vi "Configure Device.vi"(8 "error in (no error)":errorcluster, 11 "Signal Generator in":refnum<class "Signal Generator.lvclass">) -> (0 "error out":errorcluster, 3 "Signal Generator out":refnum<class "Signal Generator.lvclass">)   [LabVIEW 2020, in "Signal Generator.lvlib" / "Signal Generator.lvclass"]
uses:
  Signal Generator.lvclass
  Waveform Type.ctl
  Waveform Definition.ctl
  build/ppl/lv-hal.lvlibp/Device/Device.lvclass
  C:/dev/HAL Demo/build/ppl/lv-hal.lvlibp/Device/Device.lvclass
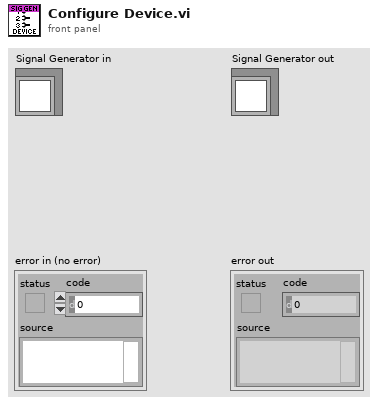
[diagram p1: front panel]
types:
  T1 = typedef "Signal Generator.lvlib/Signal Generator.lvclass/Waveform Definition.ctl" = cluster{"Waveform Type":T2, "Frequency":dbl, "Amplitude":dbl}
  T2 = typedef "Signal Generator.lvlib/Signal Generator.lvclass/Waveform Type.ctl" = enum16{"Sine Wave", "Triangle Wave", "Square Wave", "Sawtooth Wave"}
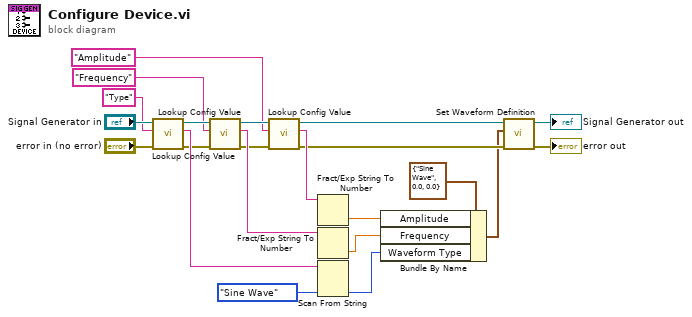
[diagram p0: block diagram]
diagram:
  n1 = call "Lookup Config Value.vi"("error in (no error)"="error in (no error)", "Config Key"="Type", "Device in"="Signal Generator in") -> ("error out"=w11:errorcluster, "Value"=w15:string, "Device out"=w19:refnum<class "Signal Generator.lvclass">)  [unwired: 5 in, 1 out]
  n2 = call "Lookup Config Value.vi"("error in (no error)"=w11, "Config Key"="Frequency", "Device in"=w19) -> ("error out"=w10:errorcluster, "Value"=w13:string, "Device out"=w17:refnum<class "Signal Generator.lvclass">)  [unwired: 5 in, 1 out]
  n3 = call "Lookup Config Value.vi"("error in (no error)"=w10, "Config Key"="Amplitude", "Device in"=w17) -> ("error out"=w8:errorcluster, "Value"=w12:string, "Device out"=w9:refnum<class "Signal Generator.lvclass">)  [unwired: 5 in, 1 out]
  n4 = Fract/Exp String To Number(string=w12) -> (number=w3:dbl)  [unwired: 3 in, 1 out]
  n5 = Fract/Exp String To Number(string=w13) -> (number=w2:dbl)  [unwired: 3 in, 1 out]
  n6 = Scan From String(input string=w15, default 1=Waveform_Type."Sine Wave" ("Waveform Type")) -> (output 1=w1:T2)  [unwired: 3 in, 3 out]
  n7 = Bundle By Name(cluster=T1 {"Waveform Type"=enum."Sine Wave", "Frequency"=0.0, "Amplitude"=0.0} ("Waveform Definition"), "Amplitude"=w3, "Frequency"=w2, "Waveform Type"=w1) -> (w4:T1)
  n8 = call "Set Waveform Definition.vi"("error in (no error)"=w8, "Waveform Definition"=w4, "Signal Generator in"=w9) -> ("error out"=→"error out":errorcluster, "Signal Generator out"=→"Signal Generator out":refnum<class "Signal Generator.lvclass">)  [unwired: 7 in]
